vi "set_speed_params.vi"(6 "pixel-dwell time":dbl[unit]=-1.0, 7 "speed param":T1(ring), 8 "error in (no error)":errorcluster, 9 "line-scan time":dbl[unit]=-1.0, 10 "frame rate":dbl[unit]=-1.0, 11 "TrajectoryMG100122AODFrameScan in":refnum<class "TrajectoryMG100122AODFrameScan.lvclass">) -> (0 "error out":errorcluster, 3 "TrajectoryMG100122AODFrameScan out":refnum<class "TrajectoryMG100122AODFrameScan.lvclass">)   [LabVIEW 2010, in "TrajectoryMG100122AODFrameScan.lvclass"]
uses:
  TrajectoryMG100122AODFrameScan.lvclass
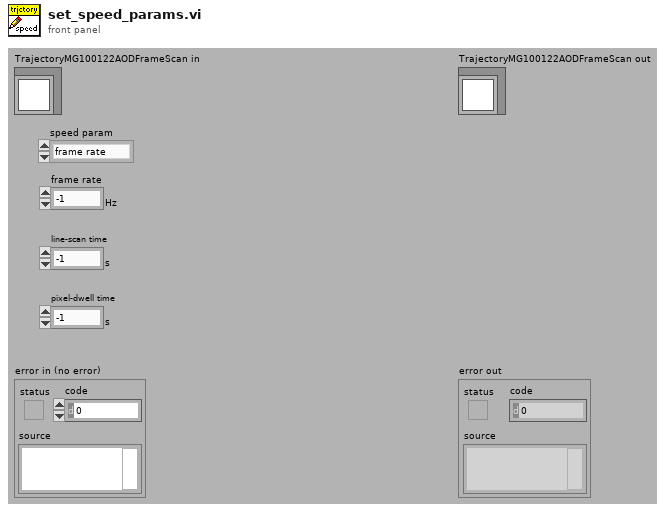
[diagram p1: front panel]
types:
  T1 = enum16{"frame rate", "line-scan time", "pixel-dwell time"}
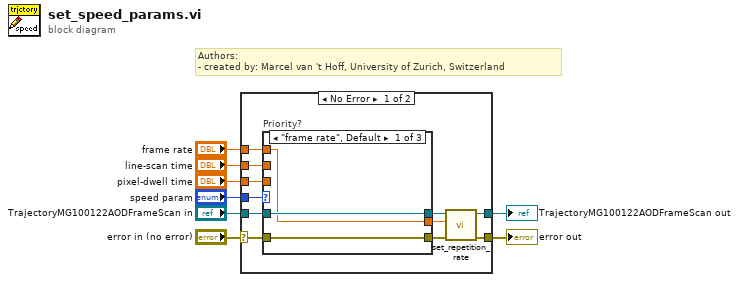
[diagram p0: block diagram]
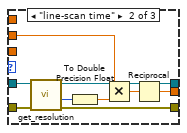
[diagram p2: hidden frame]
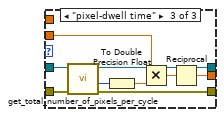
[diagram p3: hidden frame]
diagram:
  # "Authors: \n- created by: Marcel van 't Hoff, University of Zurich, Switzerland"
  n1 = case shown="No Error" "error in (no error)" {
    selector: "error in (no error)" -> [w18 w42]
    tunnel: [w14 w42] -> w7
    tunnel: [w15 w41] -> w5
    tunnel: "TrajectoryMG100122AODFrameScan in" -> [w17 w41]
    tunnel: "speed param" -> [w19 _]
    tunnel: "frame rate" -> [w12 _]
    tunnel: "line-scan time" -> [w11 _]
    tunnel: "pixel-dwell time" -> [w10 _]
    frame No Error {
      n2 = case "Priority?" shown="\"frame rate\", Default" w19 {
        tunnel: w18 -> [w22 w29 w40]
        tunnel: [w22 w28 w32] -> w13
        tunnel: [w21 w30 w33] -> w16
        tunnel: w17 -> [w21 w31 w39]
        tunnel: w12 -> [w20 _ _]
        tunnel: w11 -> [_ w25 _]
        tunnel: w10 -> [_ _ w35]
        tunnel: [w20 w23 w34] -> w9
        frame "frame rate", Default {
        }
        frame "line-scan time" {
          n3 = call-dynamic "get_resolution.vi"("error in (no error)"=w29, "TrajectoryMG100122AODFrameScan in"=w31) -> ("error out"=w28:errorcluster, "y resolution"=w24:i32, "TrajectoryMG100122AODFrameScan out"=w30:refnum<class "TrajectoryMG100122AODFrameScan.lvclass">)  [unwired: 6 in, 1 out]
          n4 = To Double Precision Float(number=w24) -> (double precision float=w26:dbl)
          n5 = Multiply(x=w25, y=w26) -> (x*y=w27:dbl[unit])
          n6 = Reciprocal(x=w27) -> (1/x=w23:dbl[unit])
        }
        frame "pixel-dwell time" {
          n7 = call-dynamic "get_total_number_of_pixels_per_cycle.vi"("error in (no error)"=w40, "TrajectoryMG100122AODFrameScan in"=w39) -> ("error out"=w32:errorcluster, "total number of pixels per cycle"=w36:i32, "TrajectoryMG100122AODFrameScan out"=w33:refnum<class "TrajectoryMG100122AODFrameScan.lvclass">)  [unwired: 7 in]
          n8 = To Double Precision Float(number=w36) -> (double precision float=w37:dbl)
          n9 = Multiply(x=w35, y=w37) -> (x*y=w38:dbl[unit])
          n10 = Reciprocal(x=w38) -> (1/x=w34:dbl[unit])
        }
      }
      n11 = call-dynamic "set_repetition_rate.vi"("error in (no error)"=w13, "repetition rate"=w9, "GenericTrajectory in"=w16) -> ("error out"=w14:errorcluster, "GenericTrajectory out"=w15:refnum<class "TrajectoryMG100122AODFrameScan.lvclass">)  [unwired: 7 in]
    }
    frame Error {
    }
  }
  "error out" <- w7
  "TrajectoryMG100122AODFrameScan out" <- w5
